vi "io_get_StatusByte.vi"(7 "Method (viReadSTB)":u16(ring) items=["viReadSTB", "*STB?"], 8 "error in":errorcluster, 10 "Bits filter (None - 0xFF)":u16=255 format="%.0x", 11 "VISA resource name":refnum<visa-resource-name>) -> (0 "error out":errorcluster, 1 "Error":bool, 2 "STB returned":u16 format="%.0x", 3 "VISA resource name out":refnum<visa-resource-name>, 4 "MAV":bool, 6 "OPC (ESB)":bool)   [LabVIEW 2014, in "rszvl_rsidr_core.lvlib"]
uses:
  rszvl_rsidr_core.lvlib
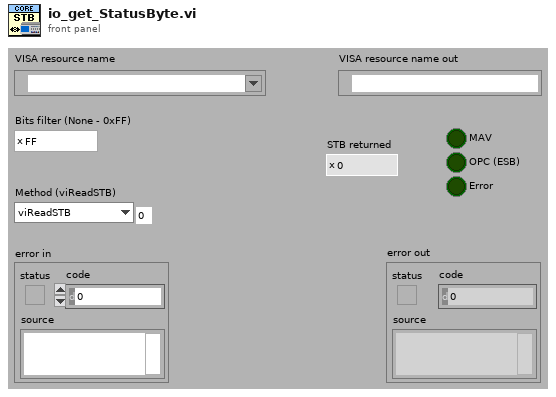
[diagram p1: front panel]
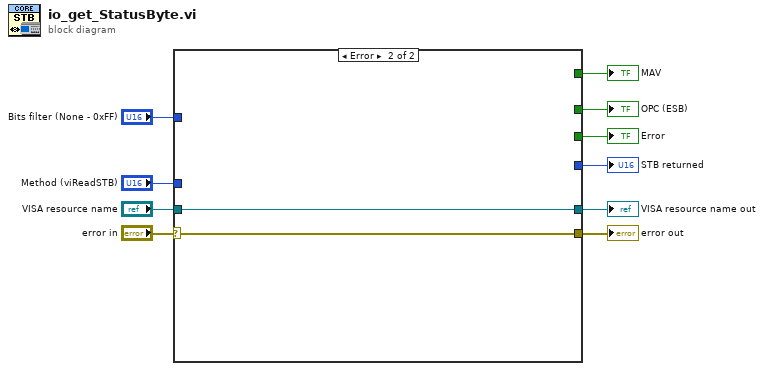
[diagram p0: block diagram]
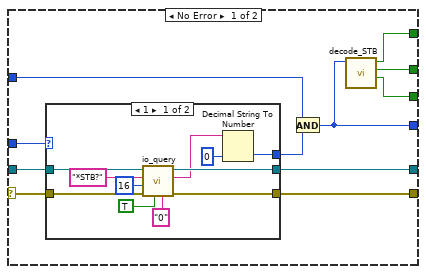
[diagram p2: hidden frame]
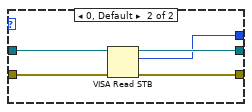
[diagram p3: hidden frame]
diagram:
  n1 = case shown="Error" "error in" {
    selector: "error in" -> [w17 w39]
    tunnel: [w21 w39] -> w10
    tunnel: "VISA resource name" -> [w18 w38]
    tunnel: [w12 _] -> w9
    tunnel: [w19 _] -> w8
    tunnel: [w15 _] -> w7
    tunnel: [w16 _] -> w6
    tunnel: [w20 w38] -> w3
    tunnel: "Method (viReadSTB)" -> [w13 _]
    tunnel: "Bits filter (None - 0xFF)" -> [w11 _]
    frame No Error {
      n2 = case shown="1" w13 {
        tunnel: [w28 w37] -> w21
        tunnel: [w27 w36] -> w20
        tunnel: w18 -> [w29 w35]
        tunnel: w17 -> [w30 w34]
        tunnel: [w31 w33] -> w14
        frame 1 {
          n3 = call "io_query.vi"("Simulation read buffer (\"Simulation\")"="0" ("Simulation read buffer \n(\"Simulation\")"), "Block Logging (F)"=TRUE, "error in"=w30, "Bytes to read (2048)"=u32 16 ("Bytes to read (1024)"), "write buffer"="*STB?", "VISA resource name"=w29) -> ("error out"=w28:errorcluster, "read buffer"=w22:string, "VISA resource name out"=w27:refnum<visa-resource-name>)  [unwired: 2 in, 1 out]
          n4 = Decimal String To Number(string=w22, default (0L)=u16 0 ("default (0 I32)")) -> (number=w31:u16)  [unwired: 1 in, 1 out]
        }
        frame 0, Default {
          n5 = VISA Read STB(8:w34, 11:w35) -> (0:w37:errorcluster, 2:w33:u16, 3:w36:refnum<visa-resource-name>)
        }
      }
      n6 = And(x=w11, y=w14) -> (x .and. y?=w12:u16)
      n7 = call "decode_STB.vi"("STB in"=w12) -> ("Error"=w15:bool, "OPC (ESB)"=w16:bool, "MAV"=w19:bool)  [unwired: 7 in, 1 out]
    }
    frame Error {
    }
  }
  "VISA resource name out" <- w3
  "error out" <- w10
  "STB returned" <- w9
  "MAV" <- w8
  "Error" <- w7
  "OPC (ESB)" <- w6
